vi "test program.vi"(0 "speed, front":cluster{dbl[], dbl[]}[](array[cluster])=[{[59.571001052856445, 59.77449989318848, 59.99300003051758, 60.21150016784668, 60.414499282836914, 60.61750030517578, 60.83650016784668, 61.05550003051758, 61.258501052856445, 61.46150016784668, 61.664499282836914, 61.86750030517578, 62.08650016784668, 62.30550003051758, 62.52400016784668, 62.74250030517578, 62.946001052856445, 63.14949989318848, 63.35249900817871, 63.57099914550781, 63.789499282836914, 63.99300003051758, 64.19649887084961, 64.41499710083008, 64.63349914550781, 64.83650207519531, 65.03950119018555, 65.2504997253418, 65.46150207519531, 65.66450119018555, 65.86800003051758, 66.08700180053711, 66.30550003051758, 66.52399826049805, 66.74300003051758, 66.94649887084961, 67.14949798583984, 67.35250091552734, 67.57100296020508, 67.78950119018555, 67.99300003051758, 68.19649887084961, 68.41499710083008, 68.63349914550781, 68.83650207519531, 69.03950119018555, 69.24300003051758, 69.44649887084961, 69.66499710083008, 69.88349914550781, 70.08650207519531, 70.28950119018555, 70.50849914550781, 70.72750091552734, 70.93050003051758, 71.13349914550781, 71.33650207519531, 71.55550003051758, 71.77449798583984, 71.97750091552734, 72.18050003051758, 72.38349914550781, 72.60250091552734, 72.8290023803711, 73.04000091552734, 73.24349975585938, 73.46200180053711, 73.68050003051758, 73.89949798583984, 74.11849975585938, 74.32149887084961, 74.52449798583984, 74.72750091552734, 74.93050003051758, 75.13349914550781, 75.33650207519531, 75.55550003051758, 75.78249740600586, 75.99349975585938, 76.21200180053711, 76.43050003051758, 76.64949798583984, 76.86849975585938, 77.07149887084961, 77.27449798583984, 77.47750091552734, 77.69600296020508, 77.91500091552734, 78.11849975585938, 78.33700180053711, 78.55550003051758, 78.75849914550781, 78.96150207519531, 79.16500091552734, 79.36849975585938, 79.58700180053711, 79.80550003051758, 80.00849914550781, 80.21150207519531, 80.43050003051758, 80.64949798583984, 80.85250091552734, 81.07100296020508, 81.29000091552734, 81.49349975585938, 81.72000122070312, 81.94649887084961, 82.14949798583984, 82.36800003051758, 82.58700180053711, 82.79050064086914, 83.00899887084961, 83.22750091552734, 83.43050003051758, 83.65699768066406, 83.88349914550781, 84.10250091552734, 84.32149887084961, 84.53999710083008, 84.75849914550781, 84.96200180053711, 85.17300033569336, 85.39949798583984, 85.61849975585938, 85.82149887084961, 86.02449798583984, 86.22750091552734, 86.44650268554688, 86.66550064086914, 86.86849975585938, 87.07149887084961], [287.36495763812997, 286.5411096528373, 275.8260023933582, 256.25288170805754, 230.76478214139743, 201.14809233549323, 167.23135232014275, 134.90340529447556, 107.78265947830646, 85.38116404534847, 68.28027050376966, 56.32963737541536, 49.405770618669564, 49.83869215008145, 55.72286894633263, 68.41883552927449, 85.3412539697124, 107.64782761089322, 134.45171344120686, 167.36706172677424, 203.45450495472983, 237.6558425142243, 271.2931354180387, 303.1602354670177, 331.5119791156222, 352.4612203546409, 368.01177954075985, 378.6669320590582, 385.40094040737245, 387.8081502127765, 388.1459770964889, 386.220028421272, 385.2405278848182, 383.52461876020607, 384.91930528506487, 388.04037626457284, 393.1693037582423, 400.92125604115176, 410.32994753765126, 424.40752679180156, 437.74164177983613, 451.82720712225563, 466.10484080590635, 482.0496179603122, 494.96526970996877, 506.3016839577267, 515.429972796934, 521.1445050614965, 521.8914826581764, 520.0131341586801, 513.0176027953916, 502.09746549824996, 486.9550961585788, 471.9062833998787, 457.7038692663052, 444.581845438604, 432.8924797016401, 423.08751696866494, 416.5852146000665, 411.73756920599124, 406.97557808753277, 401.80670794947457, 396.1761116532018, 391.6906314718911, 388.3374178662525, 386.4121502383501, 386.33615760932537, 390.1905840652787, 395.5696469634758, 403.86894554135034, 410.84053058831864, 417.65727854434874, 423.7230481520299, 427.99611250453376, 429.4149980953847, 426.5063315396821, 430.7070684102936, 426.6588125497265, 425.62534310217416, 424.3428988545502, 425.7669938190492, 428.22225832906435, 433.963755950778, 439.23509919273374, 444.8364476760478, 449.73709284172594, 452.7110219484519, 454.65475033951566, 452.5199733567778, 450.26158896197387, 438.44616383117926, 434.2763055654073, 426.8762031218957, 419.62897026016503, 410.62179594810107, 413.41020652982394, 410.8536819195035, 410.183121708652, 419.5756849153418, 429.5366260673517, 434.05306380938384, 447.8916811066776, 457.26500070924124, 467.52022473354407, 474.6161015878346, 478.90778466089154, 481.8771714237088, 480.65099382603375, 477.787191060516, 466.56028643492306, 462.84096086495725, 456.6838126060353, 446.7285350327111, 435.42663014495696, 436.6171086216056, 426.58468918478553, 420.5928464529997, 418.72389440897246, 414.7791678690206, 413.29058175587977, 412.5880056215983, 410.5665067732271, 409.0314046710356, 408.46003348202674, 406.1545665143152, 401.9719697180408, 396.30452612394794, 384.8803010004862, 368.8722802819057, 355.19058056721343, 336.12657538591094]}, {[56.18050003051758, 56.39949989318848, 56.60249900817871, 56.82099914550781, 57.039499282836914, 57.24250030517578, 57.46150016784668, 57.68050003051758, 57.883501052856445, 58.08650016784668, 58.30550003051758, 58.52449989318848, 58.72749900817871, 58.93050003051758, 59.133501052856445, 59.35200119018555, 59.571001052856445, 59.77449989318848, 59.99300003051758, 60.21150016784668, 60.414499282836914, 60.61750030517578, 60.83650016784668, 61.05550003051758, 61.258501052856445, 61.46150016784668, 61.664499282836914, 61.86750030517578, 62.08650016784668, 62.30550003051758, 62.52400016784668, 62.74250030517578, 62.946001052856445, 63.14949989318848, 63.35249900817871, 63.57099914550781, 63.789499282836914, 63.99300003051758, 64.19649887084961, 64.41499710083008, 64.63349914550781, 64.83650207519531, 65.03950119018555, 65.2504997253418, 65.46150207519531, 65.66450119018555, 65.86800003051758, 66.08700180053711, 66.30550003051758, 66.52399826049805, 66.74300003051758, 66.94649887084961, 67.14949798583984, 67.35250091552734, 67.57100296020508, 67.78950119018555, 67.99300003051758, 68.19649887084961, 68.41499710083008, 68.63349914550781, 68.83650207519531, 69.03950119018555, 69.24300003051758, 69.44649887084961, 69.66499710083008, 69.88349914550781, 70.08650207519531, 70.28950119018555, 70.50849914550781, 70.72750091552734, 70.93050003051758, 71.13349914550781, 71.33650207519531, 71.55550003051758, 71.77449798583984, 71.97750091552734, 72.18050003051758, 72.38349914550781, 72.60250091552734, 72.8290023803711, 73.04000091552734, 73.24349975585938, 73.46200180053711, 73.68050003051758, 73.89949798583984, 74.11849975585938, 74.32149887084961, 74.52449798583984, 74.72750091552734, 74.93050003051758, 75.13349914550781, 75.33650207519531, 75.55550003051758, 75.78249740600586, 75.99349975585938, 76.21200180053711, 76.43050003051758, 76.64949798583984, 76.86849975585938, 77.07149887084961, 77.27449798583984, 77.47750091552734, 77.69600296020508, 77.91500091552734, 78.11849975585938, 78.33700180053711, 78.55550003051758, 78.75849914550781, 78.96150207519531, 79.16500091552734, 79.36849975585938, 79.58700180053711, 79.80550003051758, 80.00849914550781, 80.21150207519531, 80.43050003051758, 80.64949798583984, 80.85250091552734, 81.07100296020508, 81.29000091552734, 81.49349975585938, 81.72000122070312, 81.94649887084961, 82.14949798583984, 82.36800003051758, 82.58700180053711, 82.79050064086914, 83.00899887084961, 83.22750091552734, 83.43050003051758, 83.65699768066406, 83.88349914550781, 84.10250091552734, 84.32149887084961, 84.53999710083008, 84.75849914550781, 84.96200180053711, 85.17300033569336, 85.39949798583984, 85.61849975585938, 85.82149887084961, 86.02449798583984, 86.22750091552734, 86.44650268554688, 86.66550064086914, 86.86849975585938, 87.07149887084961, 87.27449798583984, 87.47750091552734, 87.69650268554688, 87.91550064086914, 88.11849975585938, 88.32149887084961, 88.53999710083008, 88.75849914550781, 88.96200180053711, 89.16550064086914, 89.36849975585938, 89.57149887084961, 89.77449798583984, 89.97750091552734, 90.18050003051758], [135.9908328556406, 142.95691446703935, 147.86686697297668, 150.3611600421943, 151.4038682073817, 151.2816764055109, 150.87032629022403, 151.8598738776645, 155.707306259669, 163.59683469927657, 177.29022180203813, 196.55660472791746, 217.67923332723814, 239.66627643345657, 260.1818538355873, 278.24325886163115, 287.36495763812997, 286.5411096528373, 275.8260023933582, 256.25288170805754, 230.76478214139743, 201.14809233549323, 167.23135232014275, 134.90340529447556, 107.78265947830646, 85.38116404534847, 68.28027050376966, 56.32963737541536, 49.405770618669564, 49.83869215008145, 55.72286894633263, 68.41883552927449, 85.3412539697124, 107.64782761089322, 134.45171344120686, 167.36706172677424, 203.45450495472983, 237.6558425142243, 271.2931354180387, 303.1602354670177, 331.5119791156222, 352.4612203546409, 368.01177954075985, 378.6669320590582, 385.40094040737245, 387.8081502127765, 388.1459770964889, 386.220028421272, 385.2405278848182, 383.52461876020607, 384.91930528506487, 388.04037626457284, 393.1693037582423, 400.92125604115176, 410.32994753765126, 424.40752679180156, 437.74164177983613, 451.82720712225563, 466.10484080590635, 482.0496179603122, 494.96526970996877, 506.3016839577267, 515.429972796934, 521.1445050614965, 521.8914826581764, 520.0131341586801, 513.0176027953916, 502.09746549824996, 486.9550961585788, 471.9062833998787, 457.7038692663052, 444.581845438604, 432.8924797016401, 423.08751696866494, 416.5852146000665, 411.73756920599124, 406.97557808753277, 401.80670794947457, 396.1761116532018, 391.6906314718911, 388.3374178662525, 386.4121502383501, 386.33615760932537, 390.1905840652787, 395.5696469634758, 403.86894554135034, 410.84053058831864, 417.65727854434874, 423.7230481520299, 427.99611250453376, 429.4149980953847, 426.5063315396821, 430.7070684102936, 426.6588125497265, 425.62534310217416, 424.3428988545502, 425.7669938190492, 428.22225832906435, 433.963755950778, 439.23509919273374, 444.8364476760478, 449.73709284172594, 452.7110219484519, 454.65475033951566, 452.5199733567778, 450.26158896197387, 438.44616383117926, 434.2763055654073, 426.8762031218957, 419.62897026016503, 410.62179594810107, 413.41020652982394, 410.8536819195035, 410.183121708652, 419.5756849153418, 429.5366260673517, 434.05306380938384, 447.8916811066776, 457.26500070924124, 467.52022473354407, 474.6161015878346, 478.90778466089154, 481.8771714237088, 480.65099382603375, 477.787191060516, 466.56028643492306, 462.84096086495725, 456.6838126060353, 446.7285350327111, 435.42663014495696, 436.6171086216056, 426.58468918478553, 420.5928464529997, 418.72389440897246, 414.7791678690206, 413.29058175587977, 412.5880056215983, 410.5665067732271, 409.0314046710356, 408.46003348202674, 406.1545665143152, 401.9719697180408, 396.30452612394794, 384.8803010004862, 368.8722802819057, 355.19058056721343, 336.12657538591094, 311.77463964756384, 288.92029178472455, 264.71304776558253, 244.0873365513814, 228.32395309026762, 216.9891017786532, 208.31311033494032, 203.35567505084077, 199.2627534515306, 195.29718591316322, 190.60229710970154, 184.19837795094452, 177.0554914987108, 167.8421613747444, 158.0210249485431]}], 1 "Starting x":dbl, 2 "Automatic h":bool, 5 "step":dbl=0.5, 12 "Final x":dbl=800.0, 13 "Manual h":dbl) -> (4 "calculated h":dbl=12.77610535793313, 6 "histogram":cluster{dbl[], dbl[]}(graph))   [LabVIEW 2009]
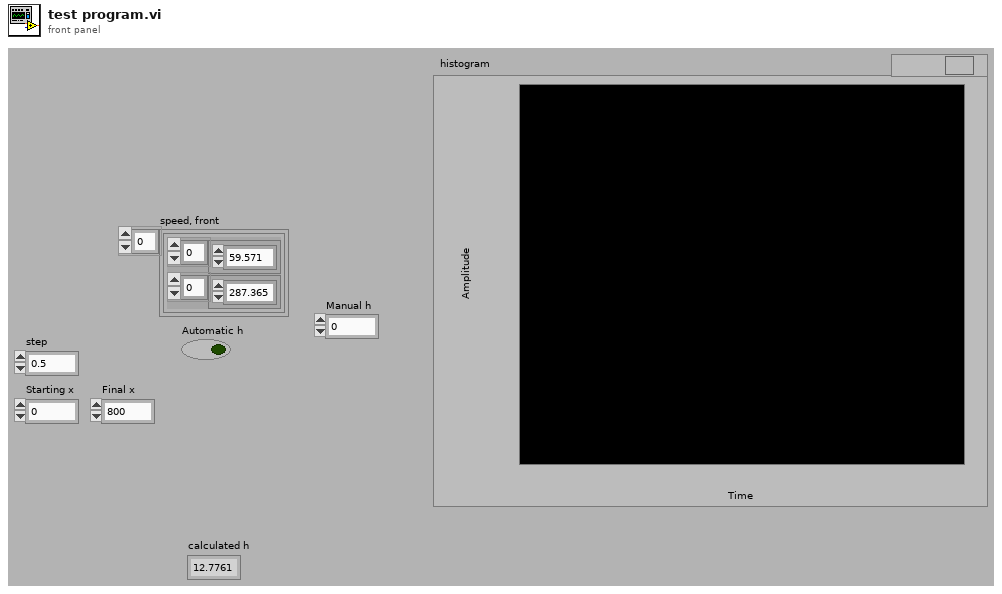
[diagram p1: front panel]
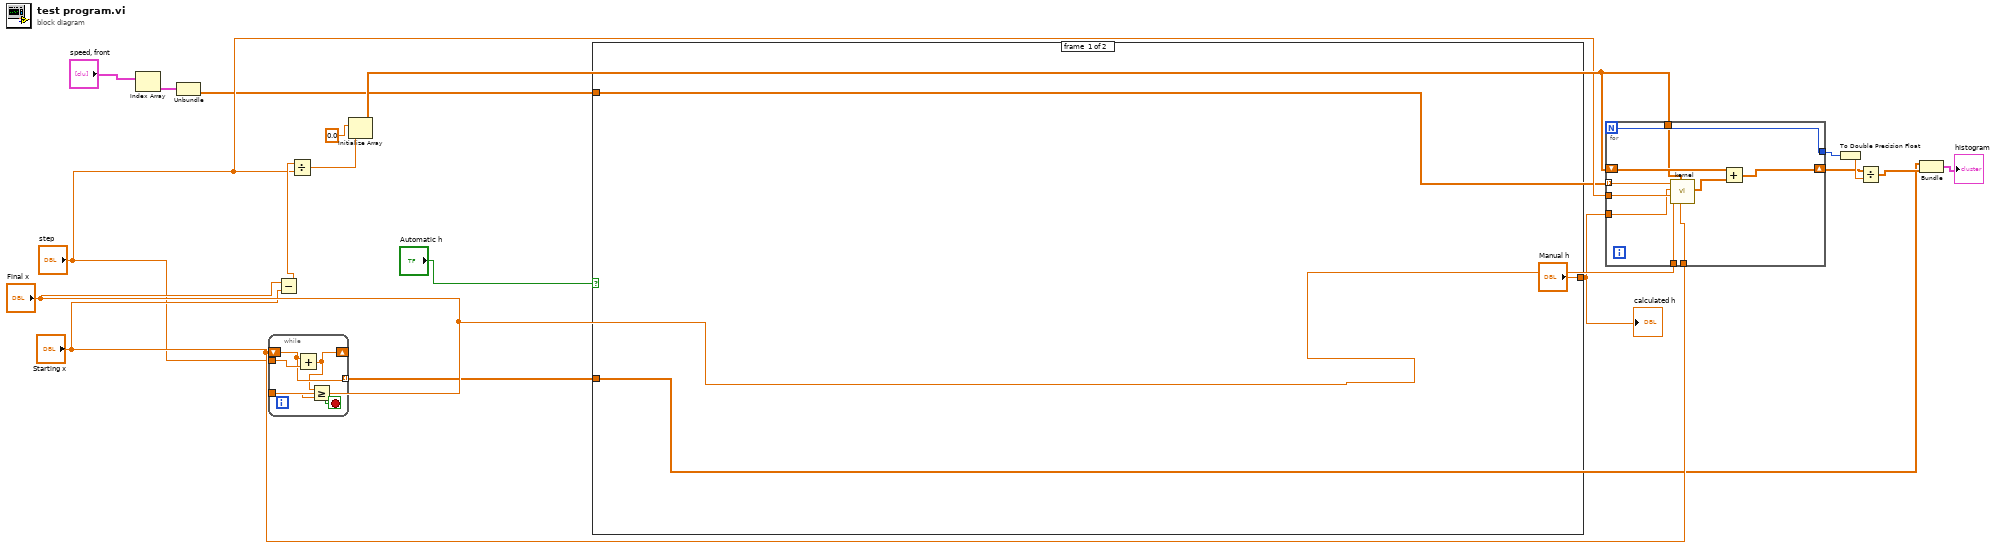
[diagram p0: block diagram]
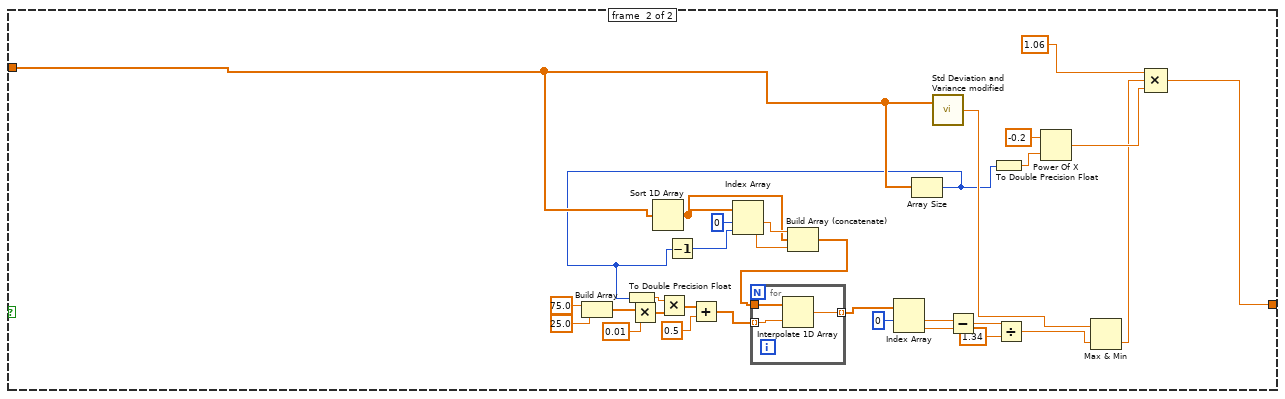
[diagram p2: hidden frame]
diagram:
  n1 = Index Array(array="speed, front") -> (element=w6:cluster{dbl[], dbl[]})  [unwired: 1 in]
  n2 = Unbundle(w6) -> (w1:dbl[])  [unwired: 1 out]
  n3 = while {
    shift-right: [w21] -> _
    shift-left: "Starting x" -> [w22]
    tunnel: "step" -> [w23]
    tunnel: [w22] -> w9 mode=indexing
    tunnel: "Final x" -> [w20]
    stop <- w19 stop-if-true
    n4 = Add(x=w22, y=w23) -> (x+y=w21:dbl)
    n5 = Greater Or Equal?(x=w21, y=w20) -> (x >= y?=w19:bool)
  }
  n6 = Subtract(x="Final x", y="Starting x") -> (x-y=w16:dbl)
  n7 = Divide(x=w16, y="step") -> (x/y=w18:dbl)
  n8 = Initialize Array(0.0 ("element"), w18) -> (w5:dbl[])
  n9 = case shown="True" "Automatic h" {
    tunnel: ["Manual h" w51] -> w2
    tunnel: w9 -> [_ _]
    tunnel: w1 -> [_ w41]
    frame #0 {
    }
    frame #1 {
      n10 = Build Array(75.0 ("element"), 25.0 ("element")) -> (w48:dbl[])
      n11 = Multiply(x=w48, y=0.01 ("element")) -> (x*y=w46:dbl[])
      n12 = Sort 1D Array(array=w41) -> (sorted array=w36:dbl[])
      n13 = Array Size(array=w41) -> (size(s)=w25:i32)
      n14 = To Double Precision Float(number=w25) -> (double precision float=w45:dbl)
      n15 = Multiply(x=w45, y=w46) -> (x*y=w44:dbl[])
      n16 = Decrement(x=w25) -> (x-1=w40:i32)
      n17 = Add(x=w44, y=0.5 ("element")) -> (x+y=w42:dbl[])
      n18 = Index Array(array=w36, index #1=0 ("index"), index #2=w40) -> (element #1=w38:dbl, element #2=w37:dbl)
      n19 = Build Array (concatenate)(w38, w36, w37) -> (w35:dbl[])
      n20 = for {
        tunnel: w42 -> [w58] mode=indexing
        tunnel: w35 -> [w57]
        tunnel: [w56] -> w34 mode=indexing
        n21 = Interpolate 1D Array(1:w58, 2:w57) -> (0:w56:dbl)
      }
      n22 = Index Array(array=w34, index #1=0 ("index")) -> (element #1=w32:dbl, element #2=w31:dbl)  [unwired: 1 in]
      n23 = call "Std Deviation and Variance modified.vi"("X"=w41) -> ("standard deviation"=w28:dbl)  [unwired: 1 in, 2 out]
      n24 = Subtract(x=w32, y=w31) -> (x-y=w30:dbl)
      n25 = To Double Precision Float(number=w25) -> (double precision float=w52:dbl)
      n26 = Divide(x=w30, y=1.34) -> (x/y=w27:dbl)
      n27 = Power Of X(1:w52, 2:-0.2 ("y")) -> (0:w55:dbl)
      n28 = Max & Min(x=w28, y=w27) -> (min(x,y)=w26:dbl)  [unwired: 1 out]
      n29 = Compound Arithmetic op=MULTIPLY(1.06, w26, w55) -> (w51:dbl)
    }
  }
  "calculated h" <- w2
  n30 = for {
    N -> [w63]
    tunnel: w1 -> [w68] mode=indexing
    tunnel: w2 -> [w60]
    tunnel: "step" -> [w67]
    tunnel: "Final x" -> [w66]
    shift-right: [w64] -> w11
    shift-left: w5 -> [w65]
    tunnel: [w63] -> w13
    tunnel: "Starting x" -> [w61]
    tunnel: w5 -> [w59]
    n31 = call "kernel.vi"("Starting x"=w61, "empty array"=w59, "Final x"=w66, "step"=w67, "h"=w60, "data point"=w68) -> ("Points"=w62:dbl[])  [unwired: 5 in]
    n32 = Add(x=w65, y=w62) -> (x+y=w64:dbl[])
  }
  n33 = To Double Precision Float(number=w13) -> (double precision float=w12:dbl)
  n34 = Divide(x=w11, y=w12) -> (x/y=w10:dbl[])
  n35 = Bundle(w9, w10) -> (→"histogram":cluster{dbl[], dbl[]})  [unwired: 1 in]
